vi "Read Safe Stop.vi"(7 "Actor in":refnum<class "Actor.lvclass">) -> (2 "Safe Stop":bool)   [LabVIEW 2025, in "jettl.lvlib"]
uses:
  jettl.lvlib
  Actor/Actor.lvclass
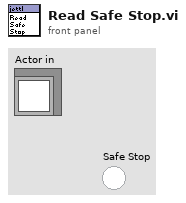
[diagram p1: front panel]
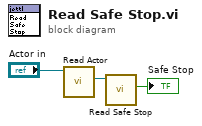
[diagram p0: block diagram]
diagram:
  n1 = call-dynamic "Read Actor.vi"("Actor in"="Actor in") -> ("Actor"=w3:refnum<class "Actor.lvclass">)  [unwired: 10 in]
  n2 = call-dynamic "Read Safe Stop.vi"("Actor in"=w3) -> ("Safe Stop"=→"Safe Stop":bool)  [unwired: 10 in]
